vi "DEMO_04_WAVE.vi"() -> ()   [LabVIEW 2014]
uses:
  <vilib>/Instr/_visa.llb/VISA Configure Serial Port (Instr).vi
panel:
  in  "打开串口":bool
  in  "上位机控制":bool
  in  "停止传送":bool
  in  "开闭环":u16(ring) items=["  开环", "  闭环"]
  in  "幅值":dbl
  in  "频率":dbl
  in  "偏移":dbl
  in  "通道选择":u16(ring) items=["一路", "二路", "三路"]
  in  "波形选择":u16(ring) items=["正弦波", "矩形波", "三角波", "锯齿波"]
  in  "发送数据":bool
  in  "波特率":u32(ring)=9600 items=["75"=75, "110"=110, "134"=134, "150"=150, "300"=300, "600"=600, "1200"=1200, "1800"=1800, "2400"=2400, "4800"=4800, "7200"=7200, "9600"=9600, "14400"=14400, "19200"=19200, "28800"=28800, "38400"=38400, "56000"=56000, "57600"=57600, "115200"=115200, "128000"=128000, "230400"=230400]
  in  "奇偶":enum16{"None", "Odd", "Even", "Mark", "Space"}(ring) caption="校验"
  in  "VISA资源名称":refnum<visa-resource-name>="COM1"
  # "发送波形"
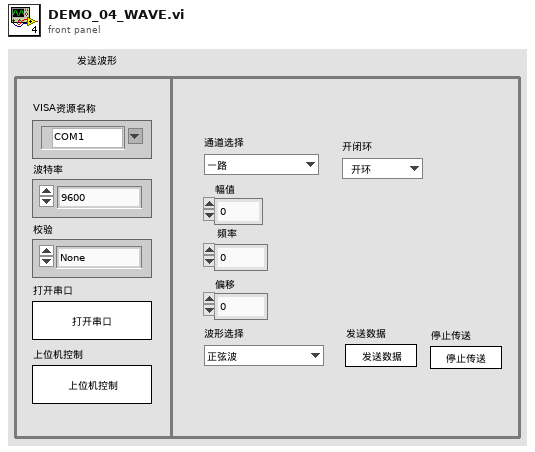
[diagram p1: front panel]
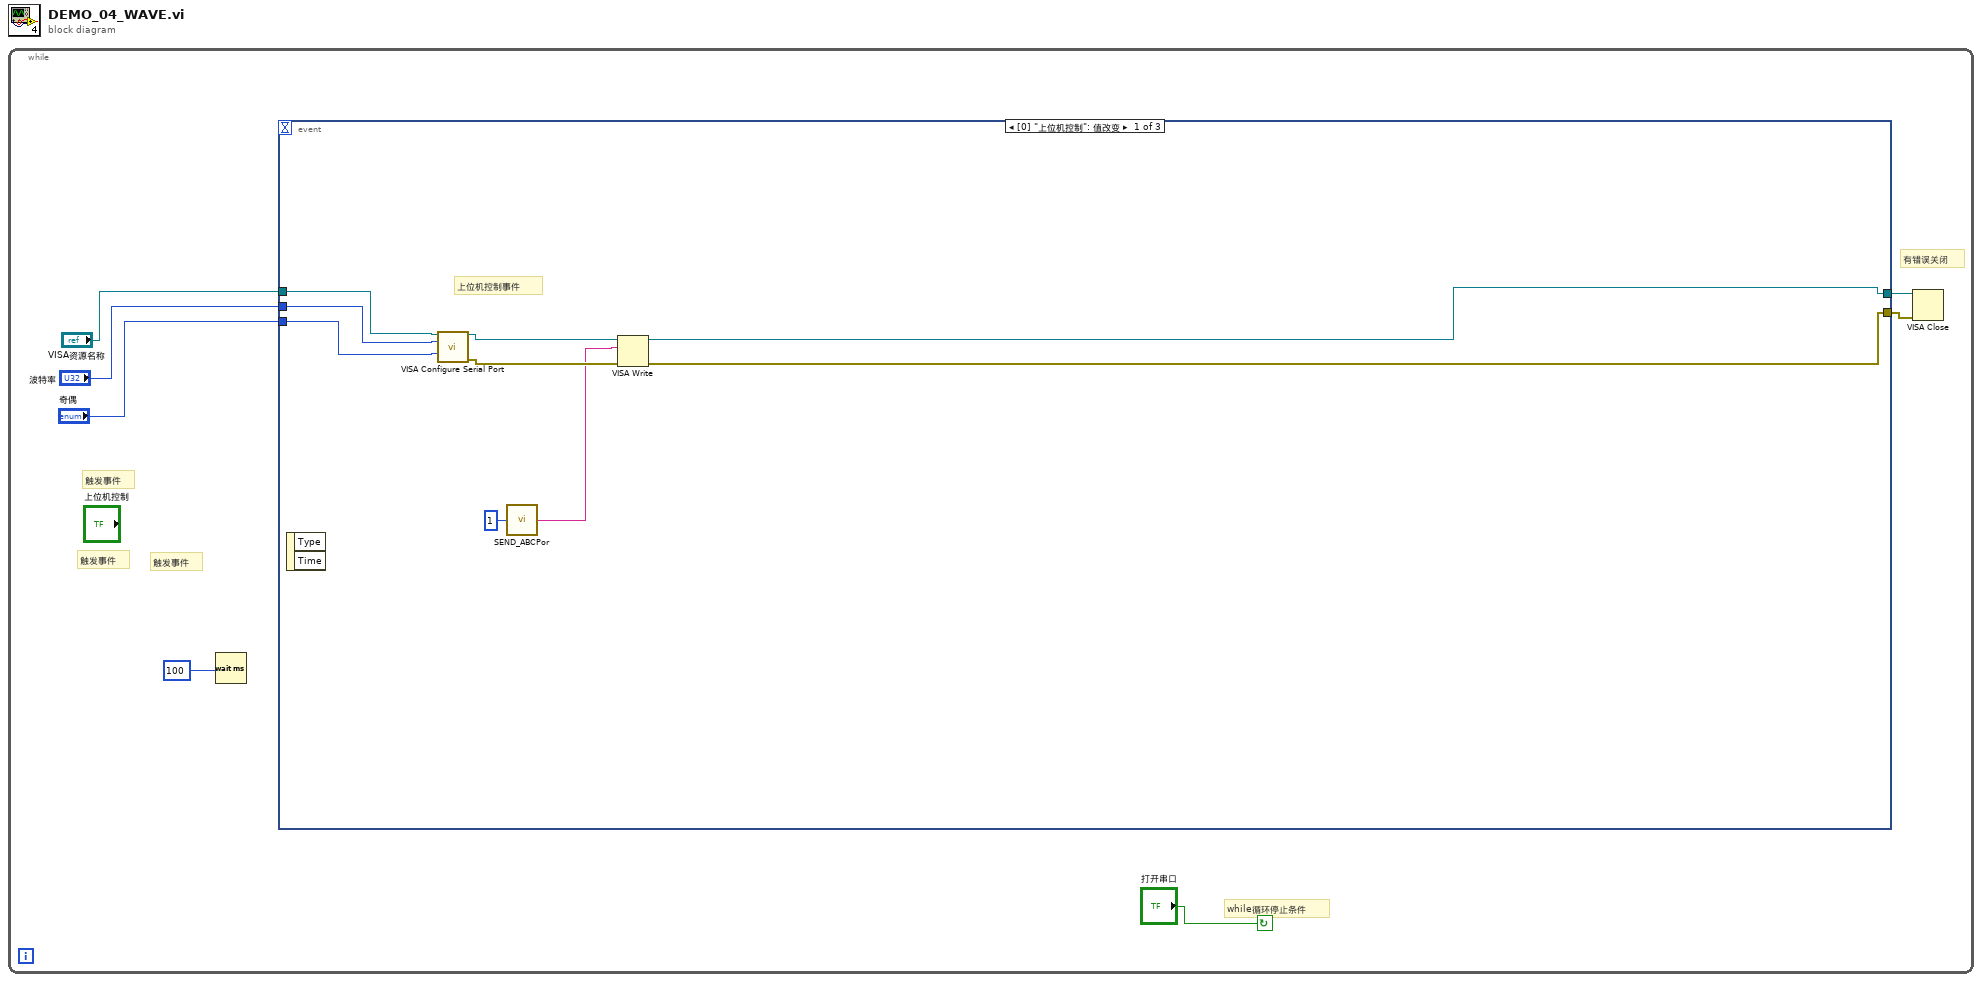
[diagram p0: block diagram]
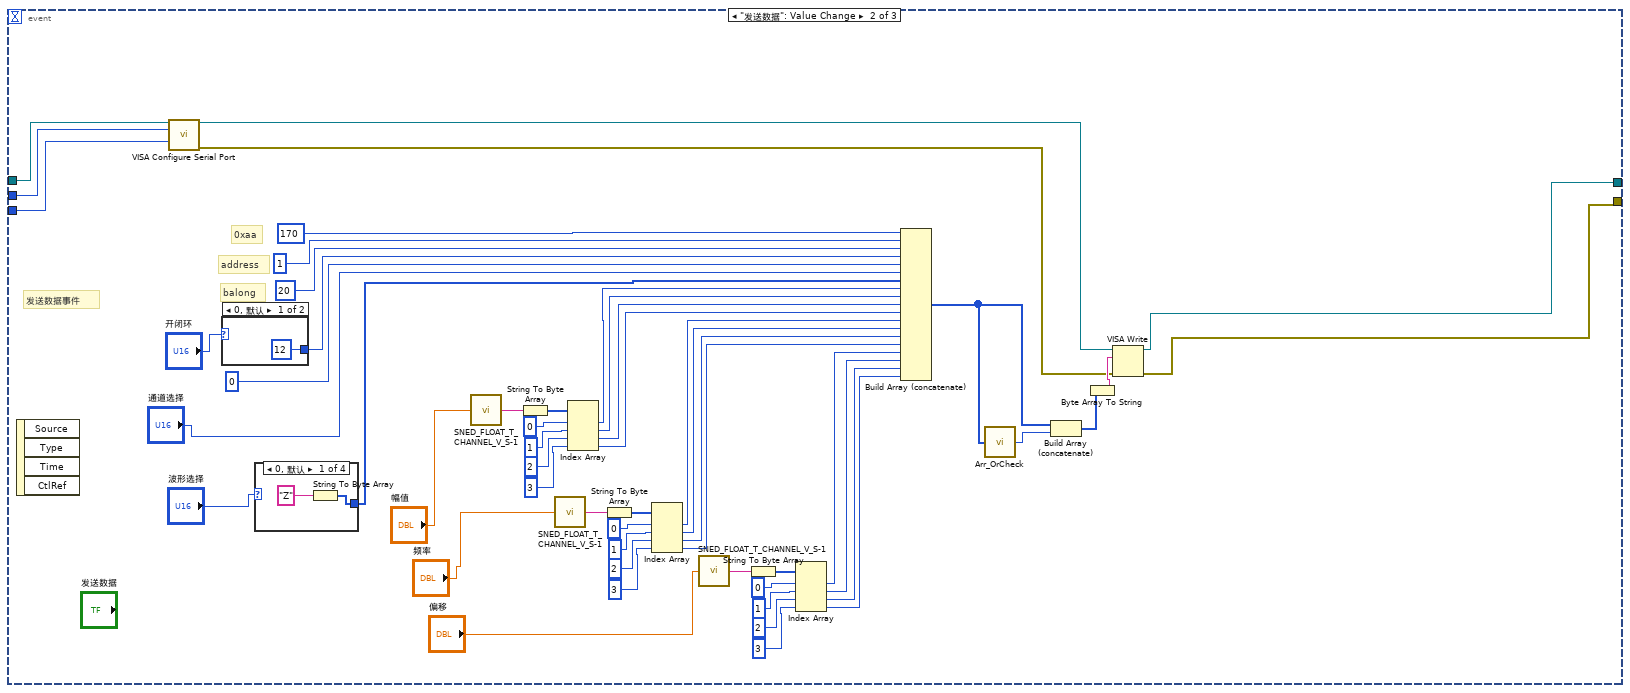
[diagram p2: hidden frame]
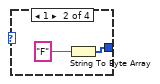
[diagram p3: hidden frame]
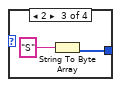
[diagram p4: hidden frame]
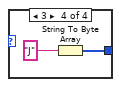
[diagram p5: hidden frame]
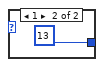
[diagram p6: hidden frame]
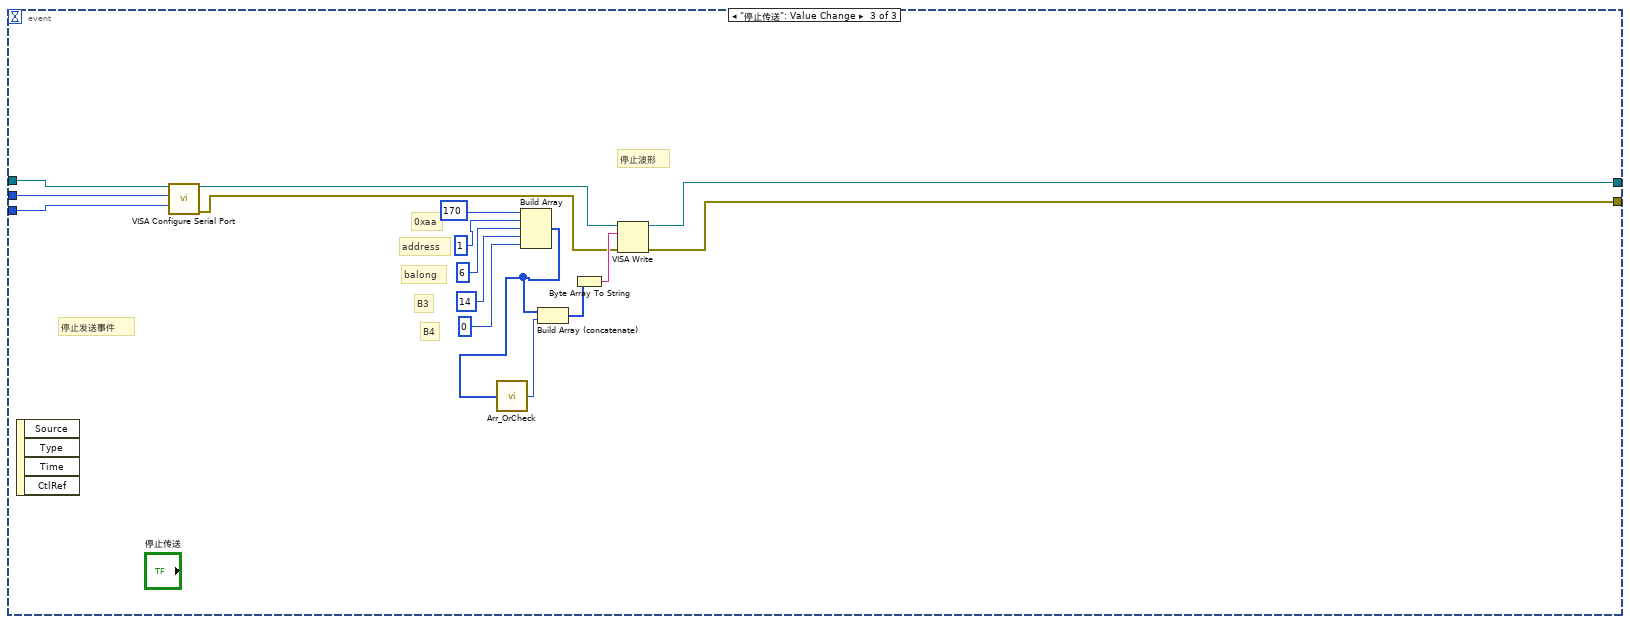
[diagram p7: hidden frame]
diagram:
  n1 = while {
    stop <- "打开串口" continue-if-true
    # "有错误关闭"
    # "while循环停止条件"
    # "触发事件"
    # "触发事件"
    # "触发事件"
    n2 = Wait (ms)(milliseconds to wait=100) -> ()  [unwired: 1 out]
    n3 = event shown="[0] \"上位机控制\": 值改变" {
      selector: _ -> [_ _ _]
      dyn-events: _ -> [_ _ _]
      timeout: _ -> [_ _ _]
      tunnel: "VISA资源名称" -> [w16 w21 w95]
      tunnel: "波特率" -> [w15 w20 w94]
      tunnel: "奇偶" -> [w14 w19 w93]
      tunnel: [w11 w23 w81] -> w2
      tunnel: [w10 w22 w80] -> w1
      event "上位机控制": Value Change {
        # "上位机控制事件"
        n4 = event-data() -> ()  [unwired: 1 in, 2 out]
        n5 = call-poly "VISA Configure Serial Port"("VISA resource name"=w16, "baud rate (9600)"=w15, "parity (0:none)"=w14) -> ("VISA resource name out"=w13:refnum<visa-resource-name>, "error out"=w12:errorcluster)  [unwired: 11 in]
        n6 = call "SEND_ABCPor.vi"("设备地址 1 开始"=1) -> ("输出字符串"=w8:string)
        n7 = VISA Write(VISA resource name=w13, write buffer=w8, error in (no error)=w12) -> (VISA resource name out=w11:refnum<visa-resource-name>, error out=w10:errorcluster)  [unwired: 1 out]
      }
      event "发送数据": Value Change {
        # "balong"
        # "address"
        # "0xaa"
        # "发送数据事件"
        n8 = event-data() -> ()  [unwired: 1 in, 4 out]
        n9 = call-poly "VISA Configure Serial Port"("VISA resource name"=w21, "baud rate (9600)"=w20, "parity (0:none)"=w19) -> ("VISA resource name out"=w25:refnum<visa-resource-name>, "error out"=w24:errorcluster)  [unwired: 11 in]
        n10 = case shown="0, 默认" "开闭环" {
          tunnel: [12 13] -> w47
          frame 0, Default {
          }
          frame 1 {
          }
        }
        n11 = case shown="0, 默认" "波形选择" {
          tunnel: [w70 w72 w74 w76] -> w45
          frame 0, Default {
            n12 = String To Byte Array(string="Z") -> (unsigned byte array=w70:u8[])
          }
          frame 1 {
            n13 = String To Byte Array(string="F") -> (unsigned byte array=w72:u8[])
          }
          frame 2 {
            n14 = String To Byte Array(string="S") -> (unsigned byte array=w74:u8[])
          }
          frame 3 {
            n15 = String To Byte Array(string="J") -> (unsigned byte array=w76:u8[])
          }
        }
        n16 = call "SNED_FLOAT_T_CHANNEL_V_S-1.vi"("数据"="幅值") -> ("字符串"=w68:string)
        n17 = String To Byte Array(string=w68) -> (unsigned byte array=w67:u8[])
        n18 = call "SNED_FLOAT_T_CHANNEL_V_S-1.vi"("数据"="频率") -> ("字符串"=w62:string)
        n19 = Index Array(array=w67, index #1=0, index #2=1, index #3=2, index #4=3) -> (element #1=w43:u8, element #2=w42:u8, element #3=w41:u8, element #4=w40:u8)
        n20 = String To Byte Array(string=w62) -> (unsigned byte array=w61:u8[])
        n21 = Index Array(array=w61, index #1=0, index #2=1, index #3=2, index #4=3) -> (element #1=w39:u8, element #2=w38:u8, element #3=w37:u8, element #4=w36:u8)
        n22 = call "SNED_FLOAT_T_CHANNEL_V_S-1.vi"("数据"="偏移") -> ("字符串"=w56:string)
        n23 = String To Byte Array(string=w56) -> (unsigned byte array=w55:u8[])
        n24 = Index Array(array=w55, index #1=0, index #2=1, index #3=2, index #4=3) -> (element #1=w35:u8, element #2=w34:u8, element #3=w33:u8, element #4=w32:u8)
        n25 = Build Array (concatenate)(170, 1, 20, w47, 0, "通道选择", w45, w43, w42, w41, w40, w39, w38, w37, w36, w35, w34, w33, w32) -> (w31:i32[])
        n26 = call "Arr_OrCheck.vi"("数组"=w31) -> ("抑或的数据值"=w30:u8)
        n27 = Build Array (concatenate)(w31, w30) -> (w29:i32[])
        n28 = Byte Array To String(unsigned byte array=w29) -> (string=w28:string)
        n29 = VISA Write(VISA resource name=w25, write buffer=w28, error in (no error)=w24) -> (VISA resource name out=w23:refnum<visa-resource-name>, error out=w22:errorcluster)  [unwired: 1 out]
      }
      event "停止传送": Value Change {
        # "停止波形"
        # "B4"
        # "B3"
        # "balong"
        # "address"
        # "0xaa"
        # "停止发送事件"
        n30 = event-data() -> ()  [unwired: 1 in, 4 out]
        n31 = call-poly "VISA Configure Serial Port"("VISA resource name"=w95, "baud rate (9600)"=w94, "parity (0:none)"=w93) -> ("VISA resource name out"=w83:refnum<visa-resource-name>, "error out"=w82:errorcluster)  [unwired: 11 in]
        n32 = Build Array(170, 1, 6, 14, 0) -> (w90:i32[])
        n33 = call "Arr_OrCheck.vi"("数组"=w90) -> ("抑或的数据值"=w89:u8)
        n34 = Build Array (concatenate)(w90, w89) -> (w91:i32[])
        n35 = Byte Array To String(unsigned byte array=w91) -> (string=w92:string)
        n36 = VISA Write(VISA resource name=w83, write buffer=w92, error in (no error)=w82) -> (VISA resource name out=w81:refnum<visa-resource-name>, error out=w80:errorcluster)  [unwired: 1 out]
      }
    }
    n37 = VISA Close(VISA resource name=w2, error in (no error)=w1) -> ()  [unwired: 1 out]
  }
